vi "CheckForErrors.vi"() -> (2 "Symbols":i32[](array[numeric]), 3 "Logs":string[][](array[string]), 4 "Paths":path[](array[path]))   [LabVIEW 2015]
doc: "Checks logs for errors"
panel:
  in  "Options":i32(listbox)
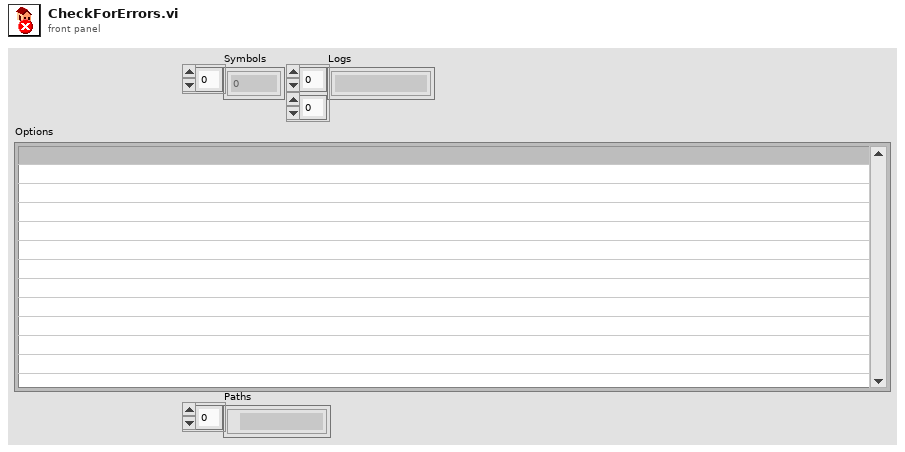
[diagram p1: front panel]
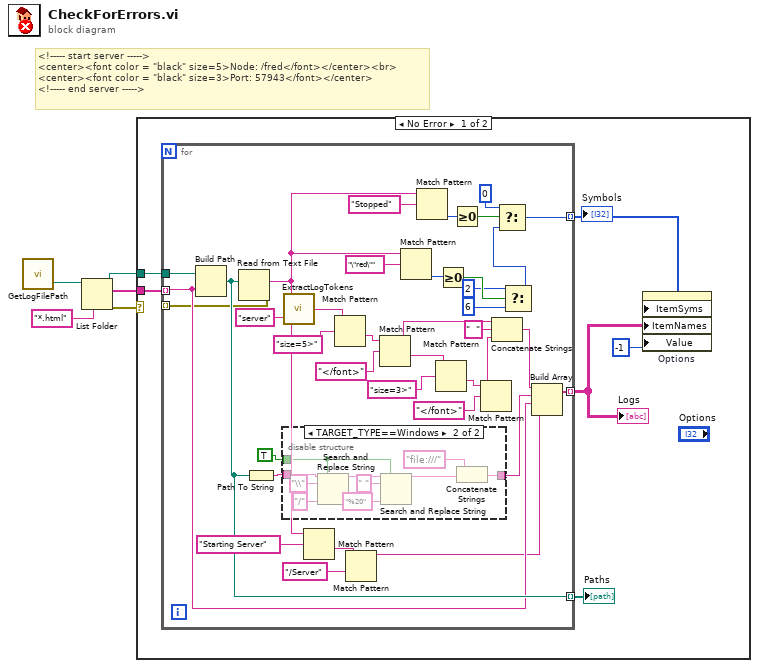
[diagram p0: block diagram]
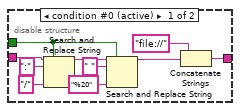
[diagram p2: hidden frame]
diagram:
  # "<!----- start server ----->\n<center><font color = \"black\" size=5>Node: /fred</font></center><br>\n<center><font color = \"black\" size=3>Port: 57943</font></center> \n<!----- end server ----->"
  n1 = call "GetLogFilePath.vi"() -> ("LogFolder"=w5:path)  [unwired: 2 in, 1 out]
  n2 = List Folder(path=w5, pattern="*.html") -> (path out=w2:path, filenames=w3:string[], error out=w1:errorcluster)  [unwired: 2 in, 1 out]
  n3 = case shown="No Error" w1 {
    tunnel: w3 -> [w11 _]
    tunnel: w2 -> [w10 _]
    frame No Error {
      n4 = for {
        tunnel: w11 -> [w19] mode=indexing
        tunnel: w10 -> [w37]
        tunnel: [w21] -> w9 mode=indexing
        tunnel: [w27] -> w7 mode=indexing
        tunnel: [w20] -> w6 mode=indexing
        tunnel: [w18] -> _ mode=indexing
        n5 = Build Path(base path=w37, name or relative path=w19) -> (appended path=w20:path)
        n6 = Read from Text File(file (use dialog)=w20) -> (text=w17:string, error out=w18:errorcluster)  [unwired: 3 in, 2 out]
        n7 = Path To String(path=w20) -> (string=w29:string)
        n8 = disable-structure shown="TARGET_TYPE==Windows" {
          disable-tunnel: TRUE ("replace all? (F)") -> [w52 w62]
          disable-tunnel: w29 -> [w53 w63]
          disable-tunnel: [w50 w59] -> w12
          frame condition #0 (active) {
            n9 = Search and Replace String(replace all?=w52, input string=w53, search string=":", replace string="/" ("replace string (\"\")")) -> (result string=w58:string)  [unwired: 4 in, 3 out]
            n10 = Search and Replace String(replace all?=w52, input string=w58, search string=" ", replace string="%20" ("replace string (\"\")")) -> (result string=w49:string)  [unwired: 4 in, 3 out]
            n11 = Concatenate Strings("file://" ("string"), w49) -> (w50:string)
          }
          frame condition #1 {
            n12 = Search and Replace String(replace all?=w62, input string=w63, search string="\\", replace string="/" ("replace string (\"\")")) -> (result string=w68:string)  [unwired: 4 in, 3 out]
            n13 = Search and Replace String(replace all?=w62, input string=w68, search string=" ", replace string="%20" ("replace string (\"\")")) -> (result string=w60:string)  [unwired: 4 in, 3 out]
            n14 = Concatenate Strings("file:///" ("string"), w60) -> (w59:string)
          }
        }
        n15 = call "ExtractLogTokens.vi"("HTML"=w17, "section"="server" ("string")) -> ("tagged text"=w47:string)  [unwired: 2 out]
        n16 = Match Pattern(string=w17, regular expression="Starting Server") -> (after substring=w16:string)  [unwired: 1 in, 3 out]
        n17 = Match Pattern(string=w47, regular expression="size=5>") -> (after substring=w45:string)  [unwired: 1 in, 3 out]
        n18 = Match Pattern(string=w16, regular expression="/Server") -> (before substring=w14:string)  [unwired: 1 in, 3 out]
        n19 = Match Pattern(string=w45, regular expression="</font>") -> (before substring=w39:string, after substring=w40:string)  [unwired: 1 in, 2 out]
        n20 = Match Pattern(string=w17, regular expression="\"red\"") -> (offset past match=w34:i32)  [unwired: 1 in, 3 out]
        n21 = Match Pattern(string=w17, regular expression="Stopped") -> (offset past match=w25:i32)  [unwired: 1 in, 3 out]
        n22 = Match Pattern(string=w40, regular expression="size=3>") -> (after substring=w42:string)  [unwired: 1 in, 3 out]
        n23 = Greater Or Equal To 0?(x=w34) -> (x >= 0?=w33:bool)
        n24 = Greater Or Equal To 0?(x=w25) -> (x >= 0?=w24:bool)
        n25 = Match Pattern(string=w42, regular expression="</font>") -> (before substring=w38:string)  [unwired: 1 in, 3 out]
        n26 = Concatenate Strings(w39, "  " ("string"), w38) -> (w28:string)
        n27 = Select(t=2, s=w33, f=6) -> (s? t:f=w22:i32)
        n28 = Select(t=0, s=w24, f=w22) -> (s? t:f=w21:i32)
        n29 = Build Array(w28, w12, w19, w14) -> (w27:string[])
      }
      "Symbols" <- w9
      "Logs" <- w7
      "Paths" <- w6
      n30 = property on="Options" class="MCListbox (strict)"("ItemSyms"=w9, "ItemNames"=w7, "Value"=-1 ("Listbox")) -> ()  [unwired: 2 in, 2 out]
    }
    frame Error {
    }
  }
